vi "FP_to_DSC.vi"(8 "error in (no error)":errorcluster, 10 "FP cluster":T1) -> (0 "error out":errorcluster)   [LabVIEW 2013]
uses:
  Typedefs/FP-cluster.ctl
  <vilib>/Platform/browser.llb/Open URL in Default Browser (string).vi
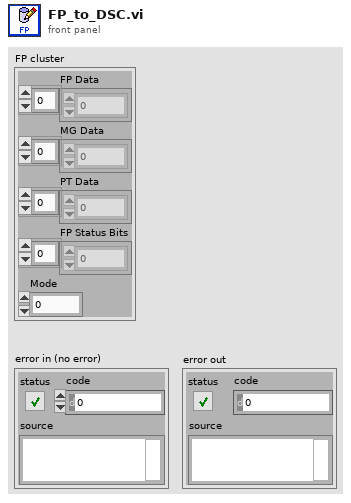
[diagram p1: front panel]
types:
  T1 = typedef "FP-cluster.ctl" = cluster{"FP Data":sgl[], "MG Data":dbl[], "PT Data":dbl[], "FP Status Bits":u32[], "Mode":u16}
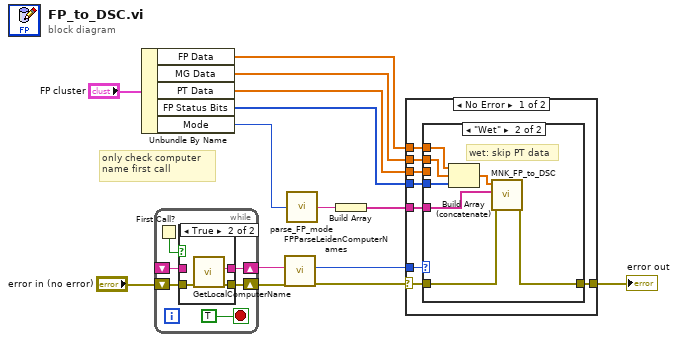
[diagram p0: block diagram]
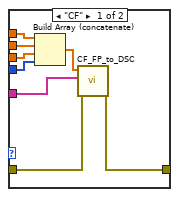
[diagram p3: hidden frame]
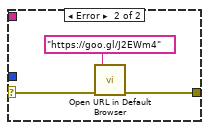
[diagram p4: hidden frame]
diagram:
  # "only check computer\nname first call"
  n1 = Unbundle By Name("FP cluster") -> ("FP Data"=w8:sgl[], "MG Data"=w7:dbl[], "PT Data"=w6:dbl[], "FP Status Bits"=w5:u32[], "Mode"=w1:u16)
  n2 = while {
    shift-right: [w19] -> w11
    shift-left: "error in (no error)" -> [w18]
    shift-right: [w20] -> w3
    shift-left: _ -> [w16]
    stop <- TRUE stop-if-true
    n3 = First Call?() -> (First Call?: T/F=w17:bool)
    n4 = case shown="True" w17 {
      tunnel: [w22 w25] -> w20
      tunnel: [w21 w24] -> w19
      tunnel: w18 -> [w21 w23]
      tunnel: w16 -> [w22 _]
      frame False {
      }
      frame True {
        n5 = call "GetLocalComputerName.vi"("error in (no error)"=w23) -> ("error out"=w24:errorcluster, "Name"=w25:string)  [unwired: 8 in, 1 out]
      }
    }
  }
  n6 = call "FPParseLeidenComputerNames.vi"("error in (no error)"=w11, "computer name"=w3) -> ("error out"=w12:errorcluster, "FP Type"=w2:enum32{"CF", "Wet"})  [unwired: 8 in]
  n7 = call "parse_FP_mode.vi"("line index"=w1) -> ("output string"=w13:string)
  n8 = Build Array(w13) -> (w14:string[])
  n9 = case shown="No Error" w12 {
    selector: w12 -> [w27 w51]
    tunnel: w14 -> [w33 _]
    tunnel: w6 -> [w32 _]
    tunnel: w7 -> [w31 _]
    tunnel: w8 -> [w30 _]
    tunnel: w5 -> [w29 _]
    tunnel: w2 -> [w28 _]
    tunnel: [w26 w50] -> w10
    frame No Error {
      n10 = case shown="\"Wet\"" w28 {
        tunnel: w30 -> [w40 w48]
        tunnel: w31 -> [w39 w47]
        tunnel: w32 -> [w38 _]
        tunnel: w33 -> [w37 w44]
        tunnel: w29 -> [w36 w46]
        tunnel: w27 -> [w35 w43]
        tunnel: [w34 w42] -> w26
        frame "CF" {
          n11 = Build Array (concatenate)(w40, w39, w38, w36) -> (w41:dbl[])
          n12 = call "CF_FP_to_DSC.vi"("error in (no error)"=w35, "str"=w37, "dbl"=w41) -> ("error out"=w34:errorcluster)  [unwired: 8 in]
        }
        frame "Wet" {
          # "wet: skip PT data"
          n13 = Build Array (concatenate)(w48, w47, w46) -> (w45:dbl[])
          n14 = call "MNK_FP_to_DSC.vi"("error in (no error)"=w43, "str"=w44, "dbl"=w45) -> ("error out"=w42:errorcluster)  [unwired: 8 in]
        }
      }
    }
    frame Error {
      n15 = call-poly <vilib>:"Open URL in Default Browser.vi"("error in (no error)"=w51, "URL"="https://goo.gl/J2EWm4") -> ("error out"=w50:errorcluster)  [unwired: 4 in, 1 out]
    }
  }
  "error out" <- w10
